vi "Auto.vi"() -> ()   [LabVIEW 2016]
panel:
  out "Sonar":dbl
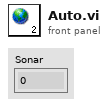
[diagram p1: front panel]
diagram:
